vi "MBUS_ModbusRead.vi"(6 "Format":u16(ring)=2 items=["Decimal", "Hexadecimal", "String"], 8 "error in":errorcluster, 9 "NumRegs":u16, 10 "StartingAddr":u16, 11 "connection ID":refnum<k5>) -> (0 "error out":errorcluster, 1 "ModbusExceptionCode":u8, 2 "outputData":u16[](array[numeric]), 3 "connection ID out":refnum<k5>, 5 "String_out":string)   [LabVIEW 2012, in "MBUS_Modbus.lvlib"]
uses:
  MBUS_Modbus.lvlib
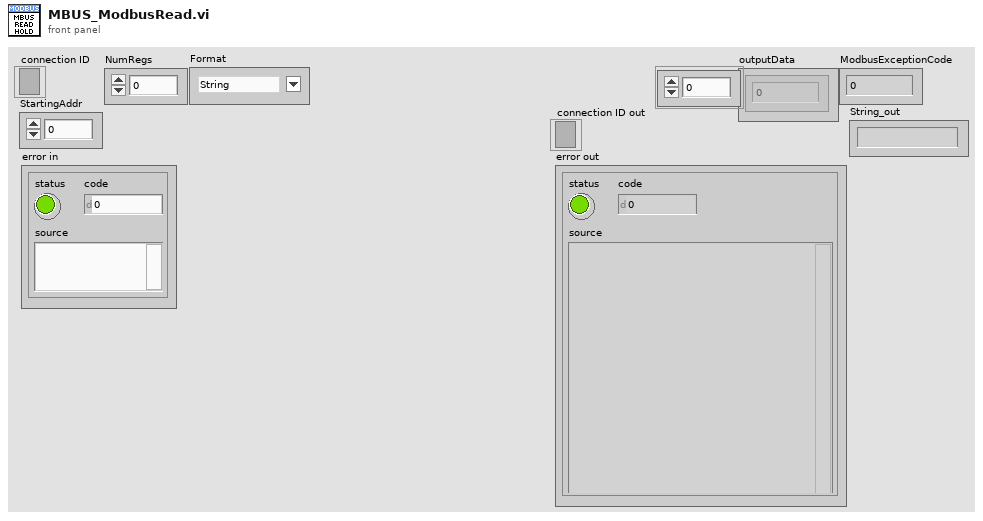
[diagram p1: front panel]
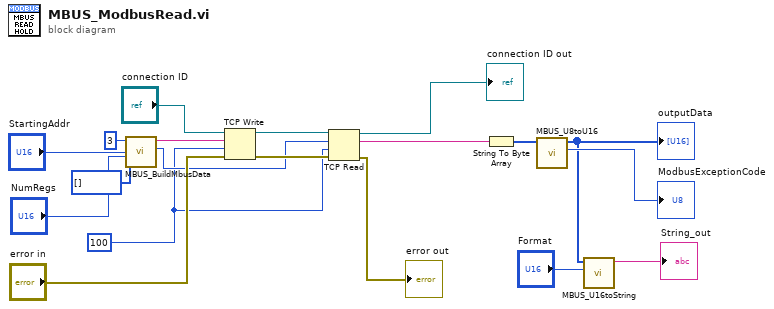
[diagram p0: block diagram]
diagram:
  w4 = 100 ("timeout ms (25000)")
  n1 = call "MBUS_BuildMbusData.vi"("data"=u16[] [], "NumRegs"="NumRegs", "StartingAddr"="StartingAddr", "MFC"=u8 3) -> ("sizeOfReturnData"=w8:u16, "dataOut"=w18:string)  [unwired: 6 in]
  n2 = TCP Write(connection ID="connection ID", data in=w18, error in (no error)="error in", 9:w4) -> (connection ID out=w19:refnum<k5>, error out=w10:errorcluster)  [unwired: 1 out]
  n3 = TCP Read(connection ID=w19, bytes to read=w8, error in (no error)=w10, 9:w4) -> (connection ID out=→"connection ID out":refnum<k5>, data out=w7:string, error out=→"error out":errorcluster)  [unwired: 1 in]
  n4 = String To Byte Array(string=w7) -> (unsigned byte array=w6:u8[])
  n5 = call "MBUS_U8toU16.vi"("inputData"=w6) -> ("ModbusExceptionCode"=→"ModbusExceptionCode":u8, "outputData"=w3:u16[])  [unwired: 9 in]
  "outputData" <- w3
  n6 = call "MBUS_U16toString.vi"("Format"="Format", "U16_in"=w3) -> ("String_out"=→"String_out":string)  [unwired: 9 in]
